vi "power_meas.vi"(0 "Input data":dbl[][](array[numeric]), 1 "Time":dbl, 2 "Voltage channel":T1, 3 "Current channel":T1, 4 "Clear Graph?":bool) -> (5 "appended array":cluster{dbl[], dbl[]}[](array[cluster]))   [LabVIEW 2016]
uses:
  INPUTS.ctl
  <vilib>/Analysis/5stat.llb/RMS (DBL).vi
  <vilib>/Analysis/NI_AALPro.lvlib
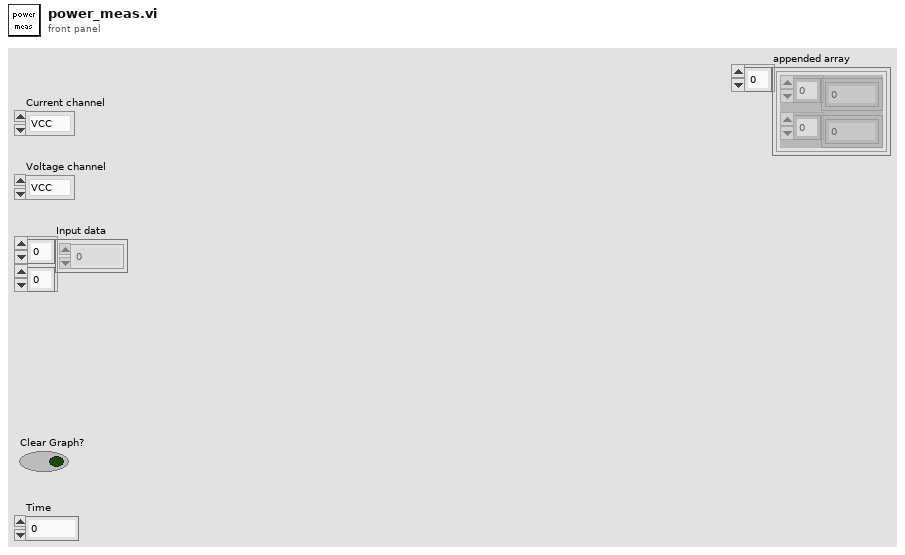
[diagram p1: front panel]
types:
  T1 = typedef "INPUTS.ctl" = enum16{"VCC", "I_PV", "I_LOAD", "I_CELL", "V_BUS", "V_CELL"}
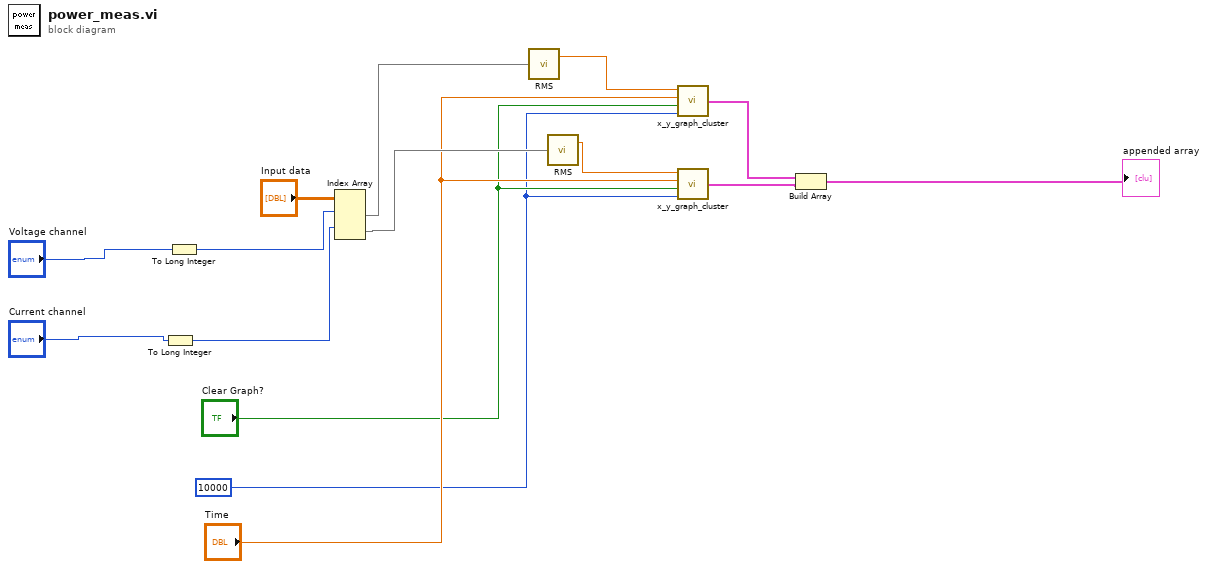
[diagram p0: block diagram]
diagram:
  w2 = 10000 ("Chart History (10,000)")
  n1 = To Long Integer(number="Current channel") -> (32bit integer=w11:i32)
  n2 = To Long Integer(number="Voltage channel") -> (32bit integer=w12:i32)
  n3 = Index Array(array="Input data", index (row) #1=w12, index (row) #2=w11) -> (element #1=w15:dbl[], element #2=w13:dbl[])  [unwired: 2 in]
  n4 = call-poly <vilib>:"RMS.vi"("X"=w15) -> ("rms value"=w8:dbl)  [unwired: 1 out]
  n5 = call-poly <vilib>:"RMS.vi"("X"=w13) -> ("rms value"=w5:dbl)  [unwired: 1 out]
  n6 = call "x_y_graph_cluster.vi"("Chart History (10,000)"=w2, "Clear Graph?"="Clear Graph?", "X"="Time", "Y"=w8) -> ("Cluster"=w7:cluster{dbl[], dbl[]})
  n7 = call "x_y_graph_cluster.vi"("Chart History (10,000)"=w2, "Clear Graph?"="Clear Graph?", "X"="Time", "Y"=w5) -> ("Cluster"=w1:cluster{dbl[], dbl[]})
  n8 = Build Array(w7, w1) -> (→"appended array":cluster{dbl[], dbl[]}[])
